vi "Real Matrix Balance.vi"(10 "job":T1=3 items=["Neither Permuted nor Scaled", "Permuted but not Scaled", "Scaled but not Permuted", "Both Permuted and Scaled"], 11 "Input Matrix":T2) -> (0 "error":i32, 1 "index high":i32, 2 "index low":i32, 3 "Balanced Matrix":T2, 4 "Scale":dbl[](array[numeric]))   [LabVIEW 2020, in "NI_AALPro.lvlib"]
doc: "Balances the general matrix <B>Input Matrix</B> to improve the accuracy of computed eigenvalues and eigenvectors. Wire data to the <B>Input Matrix</B> input to determine the polymorphic instance to use or manually select the instance."
uses:
  <vilib>/Analysis/NI_AALPro.lvlib
  <vilib>/Analysis/Matrix/Datatypes/RealMatrix.ctl
  <vilib>/Analysis/7linalg.llb/Matrix Balance Job.ctl
  <resource>/lvanlys.dll
  <vilib>/Analysis/Matrix/NI_Matrix.lvlib
panel:
  # "Real Matrix Balance"
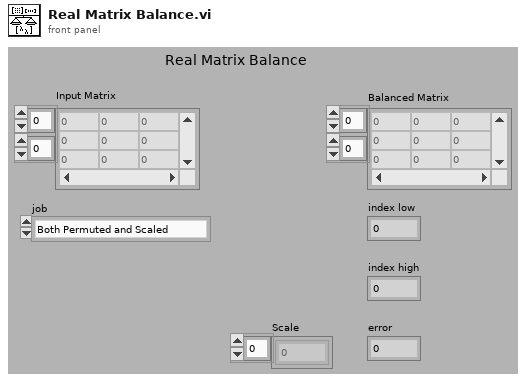
[diagram p1: front panel]
types:
  T1 = typedef "NI_AALPro.lvlib/Matrix Balance Job.ctl" = u16
  T2 = typedef "NI_Matrix.lvlib/RealMatrix.ctl" = dbl[][]
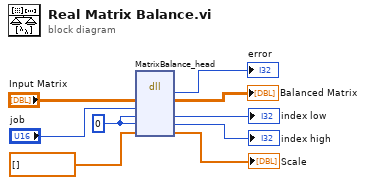
[diagram p0: block diagram]
diagram:
  w7 = 0 ("ilo")
  n1 = dll-call lib="e:/builds/penguin/labview/branches/2020/dev/dist/resource/lvanlys.*" fn="MatrixBalance_head"("Input Matrix"="Input Matrix", "job"="job", "ilo"=w7, "ihi"=w7, "output param"=dbl[] []) -> (→"error":i32, "Input Matrix"=→"Balanced Matrix":T2, "ilo"=→"index low":i32, "ihi"=→"index high":i32, "output param"=→"Scale":dbl[])  [unwired: 4 in, 2 out]
